vi "Find Owner Type.vi"(8 "Message":refnum<class "TestManagerMsg.lvclass">, 11 "Test Event Storage in":refnum<class "Test Event Storage.lvclass">) -> (0 "Message dup":refnum<class "TestManagerMsg.lvclass">, 2 "Owner Type":T1, 3 "Test Event Storage out":refnum<class "Test Event Storage.lvclass">)   [LabVIEW 2013, in "Caraya.lvlib" / "Test Event Storage.lvclass"]
uses:
  Test Event Storage.lvclass
  Store Type -- enum.ctl
  Test Manager Message/TestManagerMsg.lvclass
  Test Manager Message/TestManagerMsg.lvclass/TestManagerMsg.ctl
  Test Event Storage.lvclass/Test Event Storage.ctl
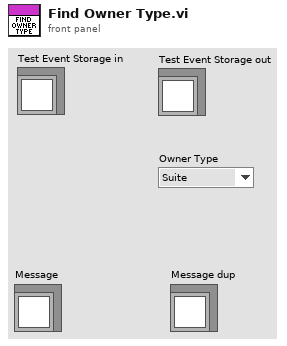
[diagram p1: front panel]
types:
  T1 = typedef "Caraya.lvlib/Test Event Storage.lvclass/Store Type -- enum.ctl" = enum16{"Suite", "Test", "Assert", "none"}
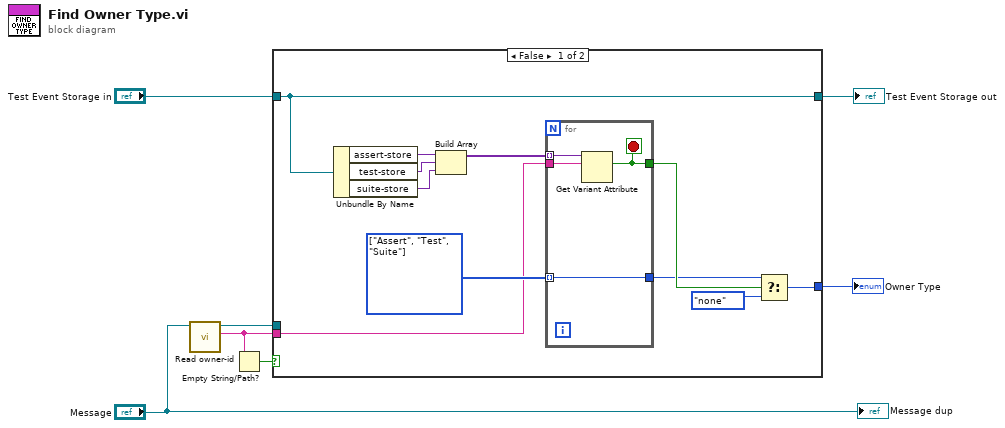
[diagram p0: block diagram]
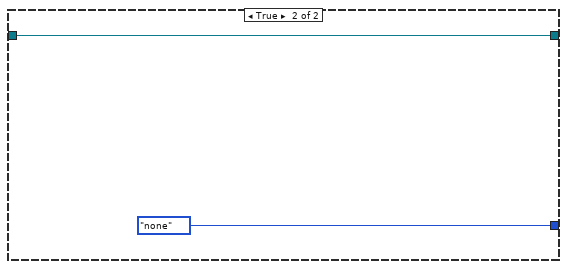
[diagram p2: hidden frame]
diagram:
  n1 = call "Read owner-id.vi"("TestManagerMsg in"="Message") -> ("owner-id"=w1:string, "TestManagerMsg out"=w2:refnum<class "TestManagerMsg.lvclass">)  [unwired: 9 in]
  n2 = Empty String/Path?(string/path=w1) -> (empty?=w3:bool)
  n3 = case shown="False" w3 {
    tunnel: "Test Event Storage in" -> [w16 w24]
    tunnel: [w17 Store_Type_--_enum."none" ("Store Type")] -> w6
    tunnel: w1 -> [w11 _]
    tunnel: w2 -> [_ _]
    tunnel: [w16 w24] -> w5
    frame False {
      w13 = T1[] [enum."Assert", enum."Test", enum."Suite"] items=["Suite", "Test", "Assert", "none"]
      n4 = Unbundle By Name(w16) -> ("assert-store"=w9:variant, "test-store"=w10:variant, "suite-store"=w8:variant)
      n5 = Build Array(w9, w10, w8) -> (w14:variant[])
      n6 = for {
        tunnel: [w20] -> w15
        tunnel: w11 -> [w22]
        tunnel: w14 -> [w21] mode=indexing
        tunnel: w13 -> [w19] mode=indexing
        tunnel: [w19] -> w12
        stop <- w20 stop-if-true
        n7 = Get Variant Attribute(Variant=w21, name=w22) -> (found=w20:bool)  [unwired: 2 in, 3 out]
      }
      n8 = Select(t=w12, s=w15, f=Store_Type_--_enum."none" ("Store Type")) -> (s? t:f=w17:T1)
    }
    frame True {
    }
  }
  "Owner Type" <- w6
  "Test Event Storage out" <- w5
  "Message dup" <- "Message"
